vi "Write Class Data.vi"(0 "System Exec Data in":refnum<class "System Exec Data.lvclass">, 1 "alias":string, 5 "standard output":string, 7 "standard error":string, 9 "return code":i32, 11 "error in (no error)":errorcluster) -> (4 "System Exec Data out":refnum<class "System Exec Data.lvclass">, 15 "error out":errorcluster)   [LabVIEW 2019, in "ProjectBuilder.lvlib" / "System Exec Data.lvclass"]
doc: "Write the status string to the private data."
uses:
  System Exec Data.lvclass
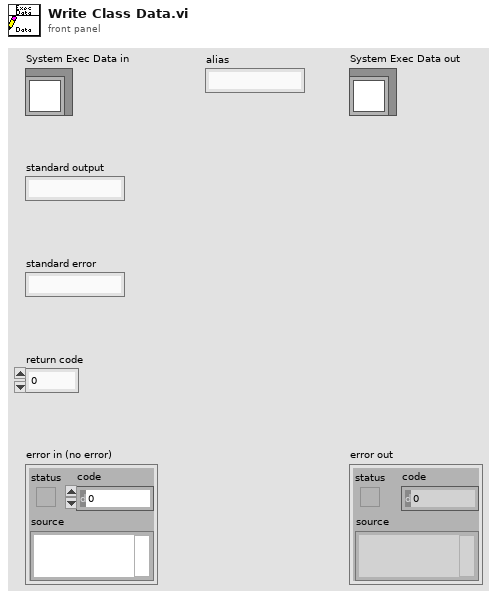
[diagram p1: front panel]
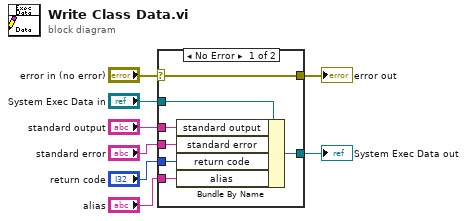
[diagram p0: block diagram]
diagram:
  n1 = case shown="No Error" "error in (no error)" {
    selector: "error in (no error)" -> [w15 w16]
    tunnel: [w15 w16] -> w7
    tunnel: [w13 w17] -> w5
    tunnel: "System Exec Data in" -> [w14 w17]
    tunnel: "standard output" -> [w12 _]
    tunnel: "standard error" -> [w11 _]
    tunnel: "return code" -> [w10 _]
    tunnel: "alias" -> [w9 _]
    frame No Error {
      n2 = Bundle By Name(cluster=w14, "standard output"=w12, "standard error"=w11, "return code"=w10, "alias"=w9) -> (w13:refnum<class "System Exec Data.lvclass">)
    }
    frame Error {
    }
  }
  "error out" <- w7
  "System Exec Data out" <- w5
